vi "Report.vi"   [LabVIEW 2014]
uses:
  g_ReportControl.vi
  g_Stop.vi
types:
  T1 = enum16{"open", "replace", "create", "open or create", "replace or create", "replace or create with confirmation"}
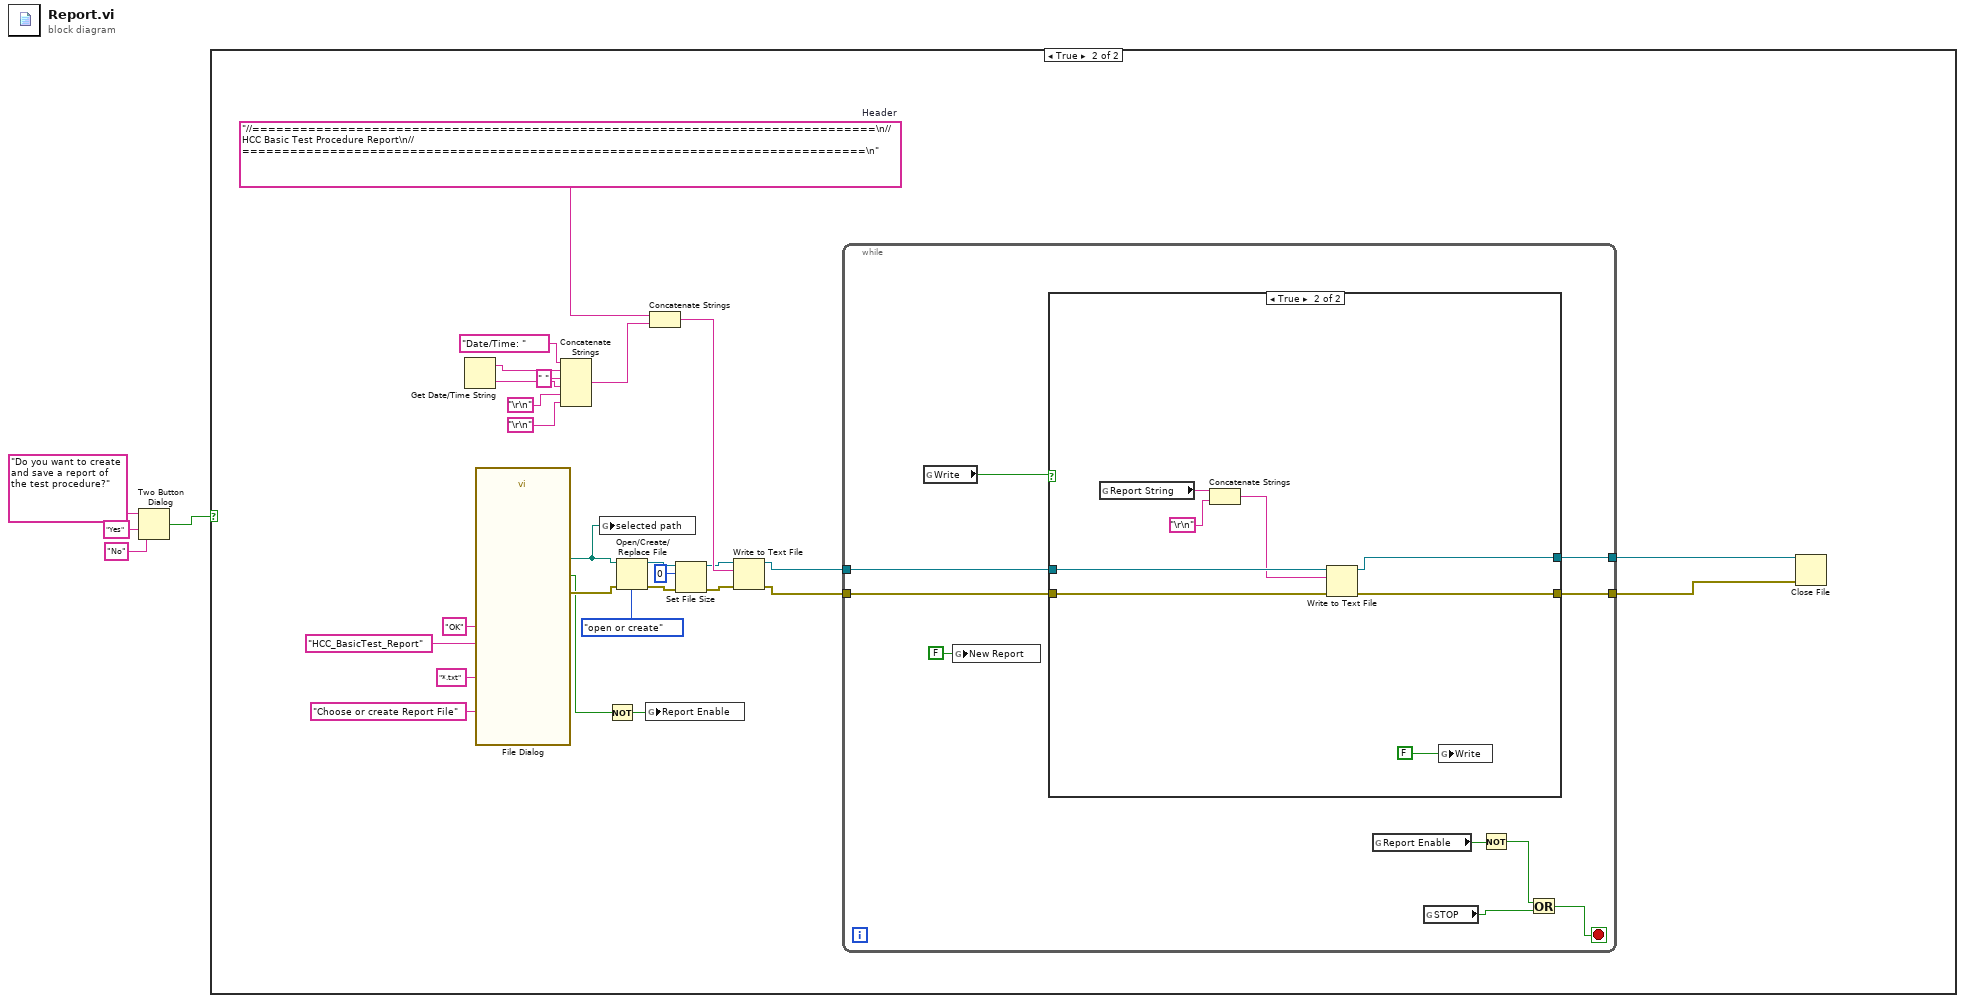
[diagram p0: block diagram]
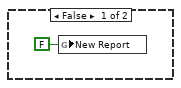
[diagram p2: hidden frame]
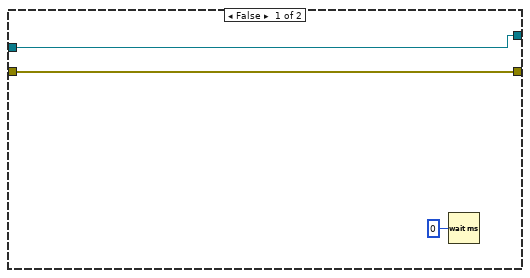
[diagram p3: hidden frame]
diagram:
  n1 = Two Button Dialog(message="Do you want to create and save a report of the test procedure?", 1:"No" ("F button name (\"Cancel\")"), 2:"Yes" ("T button name (\"OK\")")) -> (T button?=w1:bool)
  n2 = case shown="True" w1 {
    frame False {
      n3 = global write "g_ReportControl.vi" "New Report"(FALSE ("New Report")) -> ()
    }
    frame True {
      w21 = "//==============================================================================\n// HCC Basic Test Procedure Report\n//==============================================================================\n"  # Header
      n4 = Get Date/Time String() -> (date string=w26:string, time string=w25:string)  [unwired: 3 in]
      n5 = call "File Dialog"("prompt"="Choose or create Report File", "button label"="OK", "default name"="HCC_BasicTest_Report", "pattern (all files)"="*.txt") -> ("selected path"=w6:path, "cancelled"=w17:bool, "error out"=w22:errorcluster)  [unwired: 8 in, 1 out]
      n6 = Concatenate Strings("Date/Time: " ("text"), w26, " " ("string"), w25, "\r\n", "\r\n") -> (w20:string)
      n7 = global write "g_ReportControl.vi" "selected path"(w6) -> ()
      n8 = Not(x=w17) -> (.not. x?=w18:bool)
      n9 = Open/Create/Replace File(file path (use dialog)=w6, error in=w22, operation (0:open)=T1."open or create") -> (refnum out=w11:refnum<file>, error out=w10:errorcluster)  [unwired: 3 in, 1 out]
      n10 = global write "g_ReportControl.vi" "Report Enable"(w18) -> ()
      n11 = Concatenate Strings(w21, w20) -> (w19:string)
      n12 = Set File Size(4:w10, 6:i64 0 ("size (in bytes)"), 7:w11) -> (0:w9:errorcluster, 3:w8:refnum<file>)
      n13 = Write to Text File(file (use dialog)=w8, text=w19, error in=w9) -> (refnum out=w16:refnum<file>, error out=w15:errorcluster)  [unwired: 1 in, 1 out]
      n14 = while {
        tunnel: w16 -> [w40]
        tunnel: w15 -> [w39]
        tunnel: [w38] -> w14
        tunnel: [w37] -> w13
        stop <- w42 stop-if-true
        n15 = global read "g_ReportControl.vi" "Write"() -> (w41:bool)
        n16 = global write "g_ReportControl.vi" "New Report"(FALSE ("New Report")) -> ()
        n17 = case shown="True" w41 {
          tunnel: w40 -> [w45 w52]
          tunnel: w39 -> [w44 w51]
          tunnel: [w45 w50] -> w38
          tunnel: [w44 w49] -> w37
          frame False {
            n18 = Wait (ms)(milliseconds to wait=u32 0) -> ()  [unwired: 1 out]
          }
          frame True {
            n19 = global read "g_ReportControl.vi" "Report String"() -> (w48:string)
            n20 = Concatenate Strings(w48, "\r\n") -> (w47:string)
            n21 = Write to Text File(file (use dialog)=w52, text=w47, error in=w51) -> (refnum out=w50:refnum<file>, error out=w49:errorcluster)  [unwired: 1 in, 1 out]
            n22 = global write "g_ReportControl.vi" "Write"(FALSE ("Write String")) -> ()
          }
        }
        n23 = global read "g_ReportControl.vi" "Report Enable"() -> (w36:bool)
        n24 = global read "g_Stop.vi" "STOP"() -> (w34:bool)
        n25 = Not(x=w36) -> (.not. x?=w35:bool)
        n26 = Or(x=w35, y=w34) -> (x .or. y?=w42:bool)
      }
      n27 = Close File(refnum=w14, error in=w13) -> ()  [unwired: 2 out]
    }
  }
